vi "Calculate Error.vi"(8 "error in (no error)":errorcluster, 10 "ClockID":u8, 11 "Clock History Map in":T2) -> (0 "error out":errorcluster, 3 "Error Statistics (ns)":T1)   [LabVIEW 2021, in "Time_CIF_U.lvlib"]
uses:
  Time_CIF_U.lvlib
  Typedef/Clock History Map.ctl
  Typedef/Clock History.ctl
  Typedef/Timestamp Pair.ctl
  Typedef/Clock Error Statistics.ctl
  Typedef/Errors.ctl
  Errors/Append Error Location.vi
  <vilib>/Analysis/NI_AALBase.lvlib
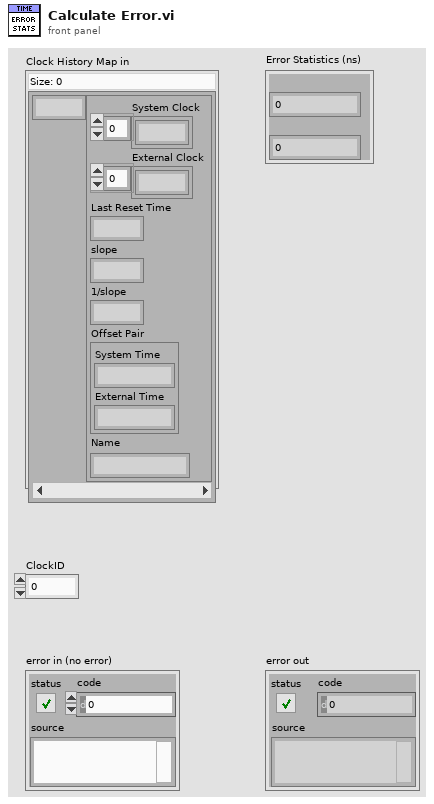
[diagram p1: front panel]
types:
  T1 = typedef "Time_CIF_U.lvlib/Clock Error Statistics.ctl" = cluster{"mean":i64, "standard deviation":i64}
  T2 = typedef "Time_CIF_U.lvlib/Clock History Map.ctl" = map{u8, T3}
  T3 = typedef "Time_CIF_U.lvlib/Clock History.ctl" = cluster{"System Clock":i64[], "External Clock":i64[], "Last Reset Time":i64, "slope":dbl, "1/slope":dbl, "Offset Pair":T4, "Name":string}
  T4 = typedef "Time_CIF_U.lvlib/Timestamp Pair.ctl" = cluster{"System Time":i64, "External Time":i64}
  T5 = typedef "Time_CIF_U.lvlib/Errors.ctl" = enum16{"Clock ID Match", "Invalid Clock ID", "Long Sleep"}
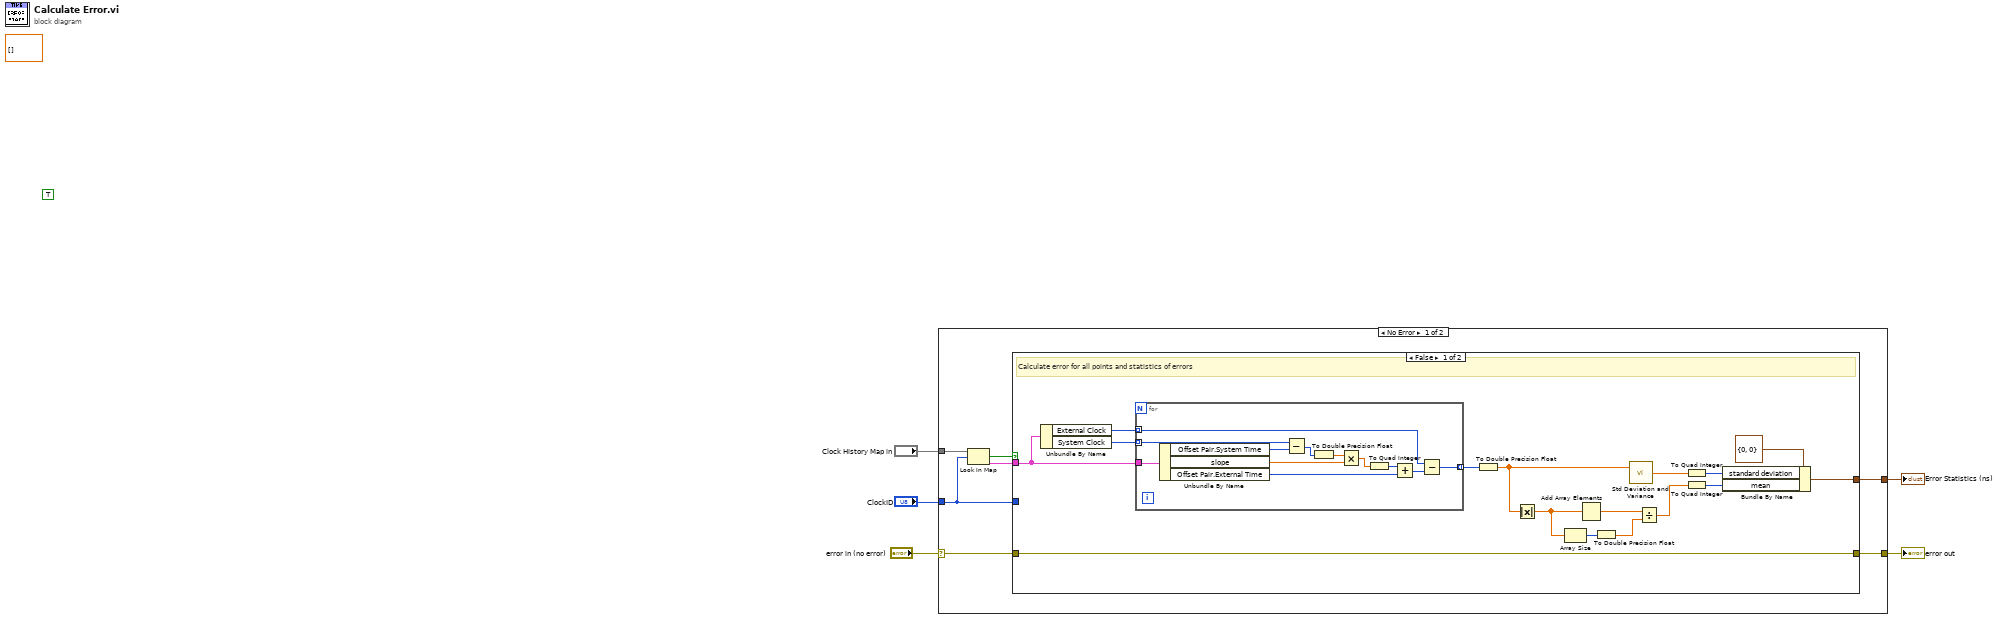
[diagram p0: block diagram]
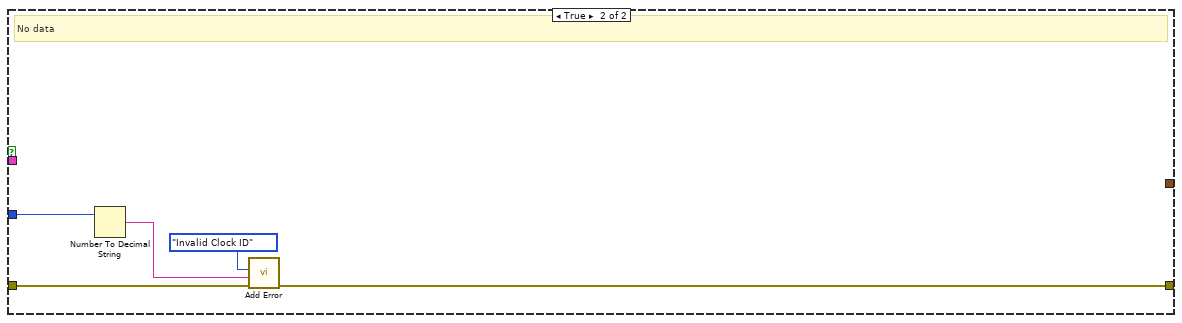
[diagram p2: hidden frame]
diagram:
  (unwired) TRUE
  (unwired) dbl[][] []
  n1 = case shown="No Error" "error in (no error)" {
    selector: "error in (no error)" -> [w10 w46]
    tunnel: "Clock History Map in" -> [w12 _]
    tunnel: [w11 w46] -> w4
    tunnel: "ClockID" -> [w6 _]
    tunnel: [w7 _] -> w1
    frame No Error {
      n2 = Look In Map(map=w12, key=w6) -> (key not found?=w8:bool, value=w9:T3)  [unwired: 1 in]
      n3 = case shown="False" w8 {
        tunnel: w9 -> [w27 _]
        tunnel: w10 -> [w28 w45]
        tunnel: [w28 w44] -> w11
        tunnel: [w13 _] -> w7
        tunnel: w6 -> [_ w41]
        frame False {
          # "Calculate error for all points and statistics of errors"
          n4 = Unbundle By Name(w27) -> ("External Clock"=w26:i64[], "System Clock"=w25:i64[])
          n5 = for {
            tunnel: w27 -> [w33]
            tunnel: w25 -> [w31] mode=indexing
            tunnel: w26 -> [w30] mode=indexing
            tunnel: [w29] -> w24 mode=indexing
            n6 = Unbundle By Name(w33) -> ("Offset Pair.System Time"=w35:i64, "slope"=w40:dbl, "Offset Pair.External Time"=w34:i64)
            n7 = Subtract(x=w31, y=w35) -> (x-y=w39:i64)
            n8 = To Double Precision Float(number=w39) -> (double precision float=w38:dbl)
            n9 = Multiply(x=w38, y=w40) -> (x*y=w37:dbl)
            n10 = To Quad Integer(1:w37) -> (0:w36:i64)
            n11 = Add(x=w36, y=w34) -> (x+y=w32:i64)
            n12 = Subtract(x=w30, y=w32) -> (x-y=w29:i64)
          }
          n13 = To Double Precision Float(number=w24) -> (double precision float=w23:dbl[])
          n14 = Absolute Value(x=w23) -> (abs(x)=w19:dbl[])
          n15 = Array Size(array=w19) -> (size(s)=w21:i32)
          n16 = Add Array Elements(numeric array=w19) -> (sum=w22:dbl)
          n17 = To Double Precision Float(number=w21) -> (double precision float=w20:dbl)
          n18 = call <vilib>:"Std Deviation and Variance.vi"("X"=w23) -> ("standard deviation"=w17:dbl)  [unwired: 1 in, 2 out]
          n19 = Divide(x=w22, y=w20) -> (x/y=w16:dbl)
          n20 = To Quad Integer(1:w17) -> (0:w15:i64)
          n21 = To Quad Integer(1:w16) -> (0:w14:i64)
          n22 = Bundle By Name(cluster=T1 {"mean"=0, "standard deviation"=0} ("Error Statistics (ns)"), "standard deviation"=w15, "mean"=w14) -> (w13:T1)
        }
        frame True {
          # "No data"
          n23 = Number To Decimal String(number=w41) -> (decimal integer string=w42:string)  [unwired: 1 in]
          n24 = call "Add Error.vi"("error in (no error)"=w45, "String to Append"=w42, "Error"=Errors."Invalid Clock ID") -> ("error out"=w44:errorcluster)  [unwired: 8 in]
        }
      }
    }
    frame Error {
    }
  }
  "error out" <- w4
  "Error Statistics (ns)" <- w1
